vi "get all FPGA CD references.vi"(8 "error in (no error)":errorcluster, 11 "Item Ref in":T1 format="%.0x") -> (0 "error out":errorcluster, 2 "RM Server refs out":T1[](array[typedef]) format="%.0x", 3 "Item Ref out":T1 format="%.0x")   [LabVIEW 2016, in "FPGA Resource Manager System Definition.lvlib"]
uses:
  FPGA Resource Manager System Definition.lvlib
  <vilib>/NI Veristand/Custom Device API/Custom Device Item Ref.ctl
  global constants.vi
  <vilib>/NI VeriStand/Custom Device API/Custom Device API.lvlib
  FPGA Resource Manager Shared.lvlib
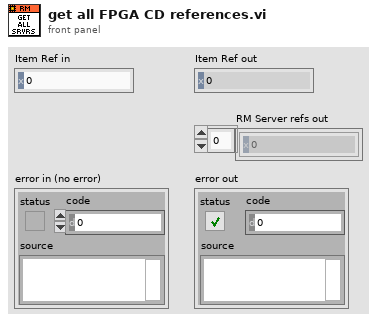
[diagram p1: front panel]
types:
  T1 = typedef "Custom Device API.lvlib/Custom Device Item Ref.ctl" = u64
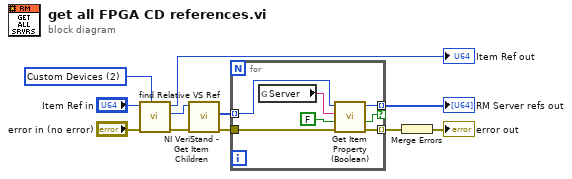
[diagram p0: block diagram]
diagram:
  w8 = u16 2 items=["Targets", "Controller", "Custom Devices", "This CD", "This CD/Group", "This CD/Group/SubGroup"] ("Relative Type")
  n1 = call "find Relative VS Ref.vi"("Relative Type"=w8, "error in (no error)"="error in (no error)", "Item Ref in"="Item Ref in") -> ("error out"=w6:errorcluster, "Relative Item Ref Out"=w10:T1, "Item Ref out"=→"Item Ref out":T1)  [unwired: 4 in, 2 out]
  n2 = call <vilib>:"NI VeriStand - Get Item Children.vi"("error in (no error)"=w6, "Item Ref in"=w10) -> ("error out"=w7:errorcluster, "Child Refs"=w11:T1[])  [unwired: 6 in, 2 out]
  n3 = for {
    tunnel: w11 -> [w18] mode=indexing
    tunnel: [w15] -> w4 mode=indexing if=w16
    tunnel: w7 -> [w13]
    tunnel: [w12] -> w3 mode=indexing
    n4 = global read "global constants.vi" "Server"() -> (w17:string)
    n5 = call <vilib>:"Get Item Property (Boolean).vi"("error in (no error)"=w13, "Default Value"=FALSE, "Property Name"=w17, "Item Ref in"=w18) -> ("error out"=w12:errorcluster, "Value"=w16:bool, "Item Ref out"=w15:T1)  [unwired: 4 in, 1 out]
  }
  "RM Server refs out" <- w4
  n6 = Merge Errors(w3) -> (→"error out":errorcluster)
